vi "DFD Filtering.vi"   [LabVIEW 2017, in "NI_DigFilterLicensed.lvlib"]
doc: "Filters an input signal continuously. Wire data to the <B>signal in</B> input to determine the polymorphic instance to use or manually select the instance."
uses:
  <vilib>/addons/Digital Filter Design/NI_DigFilterLicensed.lvlib
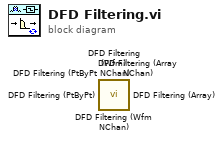
[diagram p0: block diagram]
diagram:
  n1 = call <vilib>:"DFD Filtering (Wfm NChan).vi"() -> ()  [unwired: 10 in, 2 out]
  n2 = call <vilib>:"DFD Filtering (Array NChan).vi"() -> ()  [unwired: 10 in, 2 out]
  n3 = call <vilib>:"DFD Filtering (PtByPt).vi"() -> ()  [unwired: 10 in, 2 out]
  n4 = call <vilib>:"DFD Filtering (Array).vi"() -> ()  [unwired: 10 in, 2 out]
  n5 = call <vilib>:"DFD Filtering (PtByPt NChan).vi"() -> ()  [unwired: 10 in, 2 out]
  n6 = call <vilib>:"DFD Filtering (Wfm).vi"() -> ()  [unwired: 10 in, 2 out]
